vi "RoboParser7.vi"   [LabVIEW 2015]
uses:
  GlobalVISA7.vi
  GlobalDataPointsPerPacket7.vi
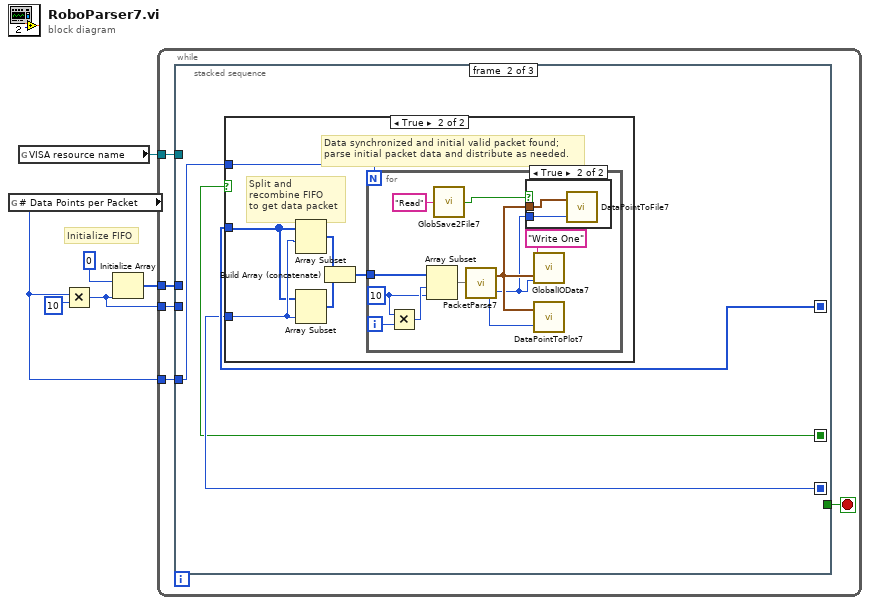
[diagram p0: block diagram]
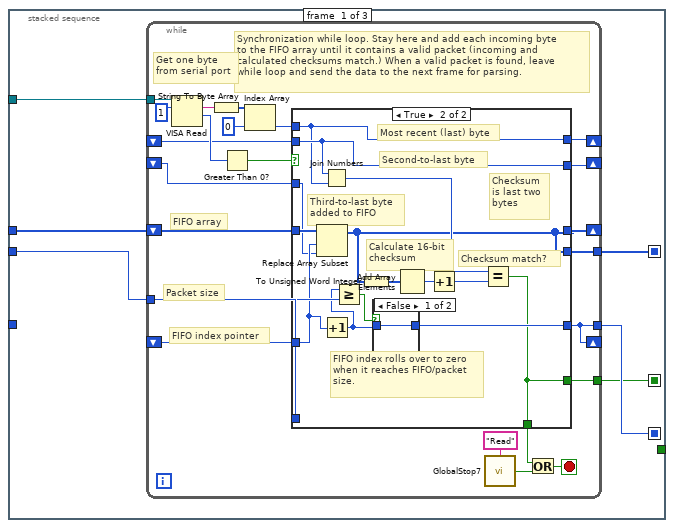
[diagram p2: hidden frame]
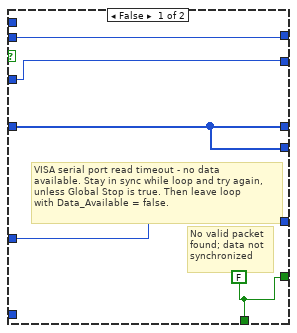
[diagram p3: hidden frame]
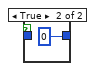
[diagram p4: hidden frame]
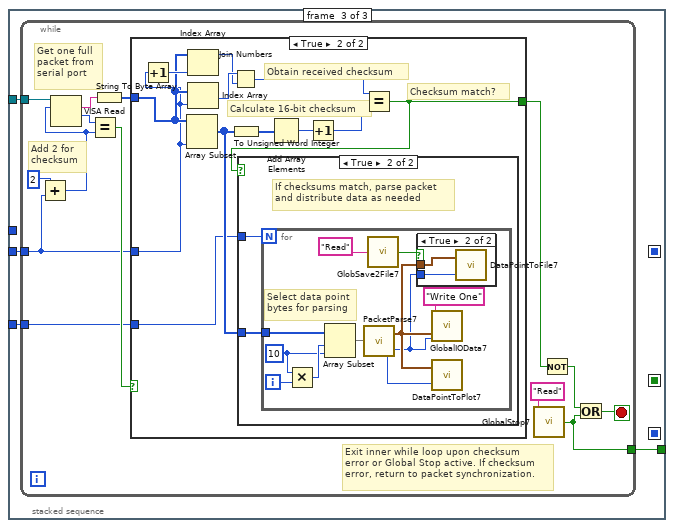
[diagram p7: hidden frame]
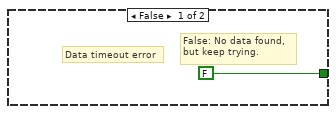
[diagram p8: hidden frame]
diagram:
  # "Initialize FIFO"
  n1 = global read "GlobalDataPointsPerPacket7.vi" "# Data Points per Packet"() -> (w1:i32)
  n2 = global read "GlobalVISA7.vi" "VISA resource name"() -> (w4:refnum<visa-resource-name>)
  n3 = Multiply(x=w1, y=10) -> (x*y=w2:i32)
  n4 = Initialize Array(u8 0, w2) -> (w5:u8[])
  n5 = while {
    tunnel: w4 -> [w9]
    tunnel: w2 -> [w11]
    tunnel: w5 -> [w10]
    tunnel: w1 -> [w7]
    stop <- w8 stop-if-true
    n6 = stacked-sequence {
      seq-local: [w14 _ _] -> [_ w66 _]
      seq-local: [w13 _ _] -> [_ w65 _]
      seq-local: [w12 _ _] -> [_ w64 _]
      tunnel: w11 -> [w17 _ w86]
      tunnel: w10 -> [w16 _ _]
      tunnel: w9 -> [w15 _ w88]
      tunnel: [_ _ w87] -> w8
      tunnel: w7 -> [_ w63 w85]
      frame #0 {
        n7 = while {
          shift-right: [w18] -> _
          shift-left: _ -> [w31]
          shift-right: [w34] -> _
          shift-left: _ -> [w32]
          tunnel: w17 -> [w30]
          shift-right: [w28] -> _
          shift-left: w16 -> [w29]
          shift-right: [w27] -> _
          shift-left: _ -> [w26]
          tunnel: w15 -> [w24]
          tunnel: [w25] -> w14
          tunnel: [w18] -> w13
          tunnel: [w23] -> w12
          stop <- w19 stop-if-true
          # "Get one byte\nfrom serial port"
          # "FIFO index pointer"
          # "Packet size"
          # "FIFO array"
          # "Synchronization while loop. Stay here and add each incoming byte\nto the FIFO array until it contains a valid packet (incoming and\ncalculated checksums match.) When a valid packet is found, leave\nwhile loop and send the data to the next frame for parsing."
          n8 = VISA Read(VISA resource name=w24, byte count=1) -> (read buffer=w39:string, return count=w36:u32)  [unwired: 1 in, 2 out]
          n9 = String To Byte Array(string=w39) -> (unsigned byte array=w38:u8[])
          n10 = Greater Than 0?(x=w36) -> (x > 0?=w35:bool)
          n11 = Index Array(array=w38, index=0) -> (element=w33:u8)
          n12 = case shown="True" w35 {
            tunnel: [w45 w51] -> w34
            tunnel: w33 -> [_ w51]
            tunnel: w32 -> [w45 w52]
            tunnel: w31 -> [w42 w57]
            tunnel: w30 -> [_ w59]
            tunnel: w29 -> [w43 w58]
            tunnel: [w43 w49] -> w28
            tunnel: [w44 w52] -> w27
            tunnel: w26 -> [w44 w56]
            tunnel: [w41 w46] -> w20
            tunnel: [w43 w49] -> w25
            tunnel: [w42 w50] -> w18
            tunnel: [w41 w46] -> w23
            frame False {
              w41 = FALSE
              # "No valid packet\nfound; data not\nsynchronized"
              # "VISA serial port read timeout - no data\navailable. Stay in sync while loop and try again,\nunless Global Stop is true. Then leave loop\nwith Data_Available = false."
            }
            frame True {
              # "FIFO index rolls over to zero\nwhen it reaches FIFO/packet\nsize."
              # "Checksum match?"
              # "Calculate 16-bit\nchecksum"
              # "Third-to-last byte\nadded to FIFO"
              # "Checksum\nis last two\nbytes"
              # "Second-to-last byte"
              # "Most recent (last) byte"
              n13 = Replace Array Subset(array=w58, new element=w56, index=w57) -> (w49:u8[])
              n14 = Join Numbers(hi=w52, lo=w51) -> ((hi.lo)=w54:u16)
              n15 = Increment(x=w57) -> (x+1=w47:i32)
              n16 = Greater Or Equal?(x=w47, y=w59) -> (x >= y?=w60:bool)
              n17 = To Unsigned Word Integer(number=w49) -> (unsigned 16bit integer=w48:u16[])
              n18 = case shown="False" w60 {
                tunnel: w47 -> [w61 _]
                tunnel: [w61 0] -> w50
                frame False {
                }
                frame True {
                }
              }
              n19 = Add Array Elements(numeric array=w48) -> (sum=w55:u16)
              n20 = Increment(x=w55) -> (x+1=w53:u16)
              n21 = Equal?(x=w54, y=w53) -> (x = y?=w46:bool)
            }
          }
          n22 = call "GlobalStop7.vi"("Function select"="Read") -> ("stop"=w21:bool)
          n23 = Or(x=w20, y=w21) -> (x .or. y?=w19:bool)
        }
      }
      frame #1 {
        n24 = case shown="True" w64 {
          tunnel: w66 -> [_ w68]
          tunnel: w65 -> [_ w69]
          tunnel: w63 -> [_ w67]
          frame False {
            # "No valid packet found, but previous while loop exited anyway.\nThis should only happen when Global Stop is activated.\nDo not parse data."
          }
          frame True {
            # "Split and \nrecombine FIFO \nto get data packet"
            # "Data synchronized and initial valid packet found;\nparse initial packet data and distribute as needed."
            n25 = Array Subset(array=w68, index=w69) -> (w72:u8[])  [unwired: 1 in]
            n26 = Array Subset(array=w68, length=w69) -> (w71:u8[])  [unwired: 1 in]
            n27 = Build Array (concatenate)(w72, w71) -> (w70:u8[])
            n28 = for {
              N: w67 -> [_]
              tunnel: w70 -> [w78]
              i -> [w82]
              w79 = 10
              n29 = Multiply(x=w79, y=w82) -> (x*y=w80:i32)
              n30 = Array Subset(array=w78, index=w80, length=w79) -> (w77:u8[])
              n31 = call "GlobSave2File7.vi"("Function select"="Read") -> ("stop"=w73:bool)
              n32 = call "PacketParse7.vi"("Packet array in"=w77) -> ("Data Point"=w76:cluster{"time":u32, "value":sgl}, "Data ID"=w75:u32)
              n33 = case shown="True" w73 {
                tunnel: w76 -> [_ w84]
                tunnel: w75 -> [_ w83]
                frame False {
                }
                frame True {
                  n34 = call "DataPointToFile7.vi"("Data ID in"=w83, "Cluster"=w84) -> ()
                }
              }
              n35 = call "GlobalIOData7.vi"("Function select"="Write One", "IO data point  in"=w76, "IO Data ID"=w75) -> ()  [unwired: 2 in, 2 out]
              n36 = call "DataPointToPlot7.vi"("Data ID in"=w75, "Cluster"=w76) -> ()
            }
          }
        }
      }
      frame #2 {
        n37 = while {
          tunnel: w88 -> [w99]
          tunnel: [w96] -> w87
          tunnel: w86 -> [w90]
          tunnel: w85 -> [w92]
          stop <- w97 stop-if-true
          # "Add 2 for\nchecksum"
          # "Exit inner while loop upon checksum\nerror or Global Stop active. If checksum\nerror, return to packet synchronization."
          # "Get one full\npacket from\nserial port"
          n38 = Add(x=2, y=w90) -> (x+y=w89:i32)
          n39 = VISA Read(VISA resource name=w99, byte count=w89) -> (read buffer=w102:string, return count=w93:u32)  [unwired: 1 in, 2 out]
          n40 = Equal?(x=w93, y=w89) -> (x = y?=w100:bool)
          n41 = String To Byte Array(string=w102) -> (unsigned byte array=w101:u8[])
          n42 = case shown="True" w100 {
            tunnel: w101 -> [_ w111]
            tunnel: [FALSE w106] -> w95
            tunnel: w90 -> [_ w105]
            tunnel: w92 -> [_ w104]
            frame False {
              # "False: No data found,\nbut keep trying."
              # "Data timeout error"
            }
            frame True {
              # "Checksum match?"
              # "Obtain received checksum"
              # "Calculate 16-bit checksum"
              n43 = Increment(x=w105) -> (x+1=w114:i32)
              n44 = Array Subset(array=w111, length=w105) -> (w107:u8[])  [unwired: 1 in]
              n45 = Index Array(array=w111, index=w114) -> (element=w112:u8)
              n46 = Index Array(array=w111, index=w105) -> (element=w113:u8)
              n47 = Join Numbers(hi=w113, lo=w112) -> ((hi.lo)=w110:u16)
              n48 = To Unsigned Word Integer(number=w107) -> (unsigned 16bit integer=w115:u16[])
              n49 = Add Array Elements(numeric array=w115) -> (sum=w109:u16)
              n50 = Increment(x=w109) -> (x+1=w108:u16)
              n51 = Equal?(x=w110, y=w108) -> (x = y?=w106:bool)
              n52 = case shown="True" w106 {
                tunnel: w107 -> [_ w117]
                tunnel: w104 -> [_ w116]
                frame False {
                  # "Invalid packet, do not parse"
                }
                frame True {
                  # "If checksums match, parse packet\nand distribute data as needed"
                  n53 = for {
                    N: w116 -> [_]
                    tunnel: w117 -> [w123]
                    i -> [w127]
                    w124 = 10
                    # "Select data point\nbytes for parsing"
                    n54 = Multiply(x=w124, y=w127) -> (x*y=w125:i32)
                    n55 = Array Subset(array=w123, index=w125, length=w124) -> (w122:u8[])
                    n56 = call "PacketParse7.vi"("Packet array in"=w122) -> ("Data Point"=w121:cluster{"time":u32, "value":sgl}, "Data ID"=w120:u32)
                    n57 = call "GlobSave2File7.vi"("Function select"="Read") -> ("stop"=w118:bool)
                    n58 = case shown="True" w118 {
                      tunnel: w121 -> [_ w129]
                      tunnel: w120 -> [_ w128]
                      frame False {
                      }
                      frame True {
                        n59 = call "DataPointToFile7.vi"("Data ID in"=w128, "Cluster"=w129) -> ()
                      }
                    }
                    n60 = call "GlobalIOData7.vi"("Function select"="Write One", "IO data point  in"=w121, "IO Data ID"=w120) -> ()  [unwired: 2 in, 2 out]
                    n61 = call "DataPointToPlot7.vi"("Data ID in"=w120, "Cluster"=w121) -> ()
                  }
                }
              }
            }
          }
          n62 = call "GlobalStop7.vi"("Function select"="Read") -> ("stop"=w96:bool)
          n63 = Not(x=w95) -> (.not. x?=w94:bool)
          n64 = Or(x=w94, y=w96) -> (x .or. y?=w97:bool)
        }
      }
    }
  }
